vi "PixelLIDAR_Open.vi"() -> (2 "error out":errorcluster, 3 "initialized LIDAR\narray":i32[](array[numeric]), 4 "MDF Image":T1(plugin-control), 5 "MissionMap":path)   [LabVIEW 2012]
doc: "This SubVI sets up the memory space for the Lidars's MDF file and reads the MDF file into it. It is designed to run before Pixel_LIDAR_Run.VI."
panel:
  out "concatenated string":string
  out "Current Path Name":string
  out "Y Resolution":i32
  out "X Resolution":i32
  # "This SubVI is used with PixelLIDAR_Run.VI and reads thw Mission Map file and sets up memory to accomidate it"
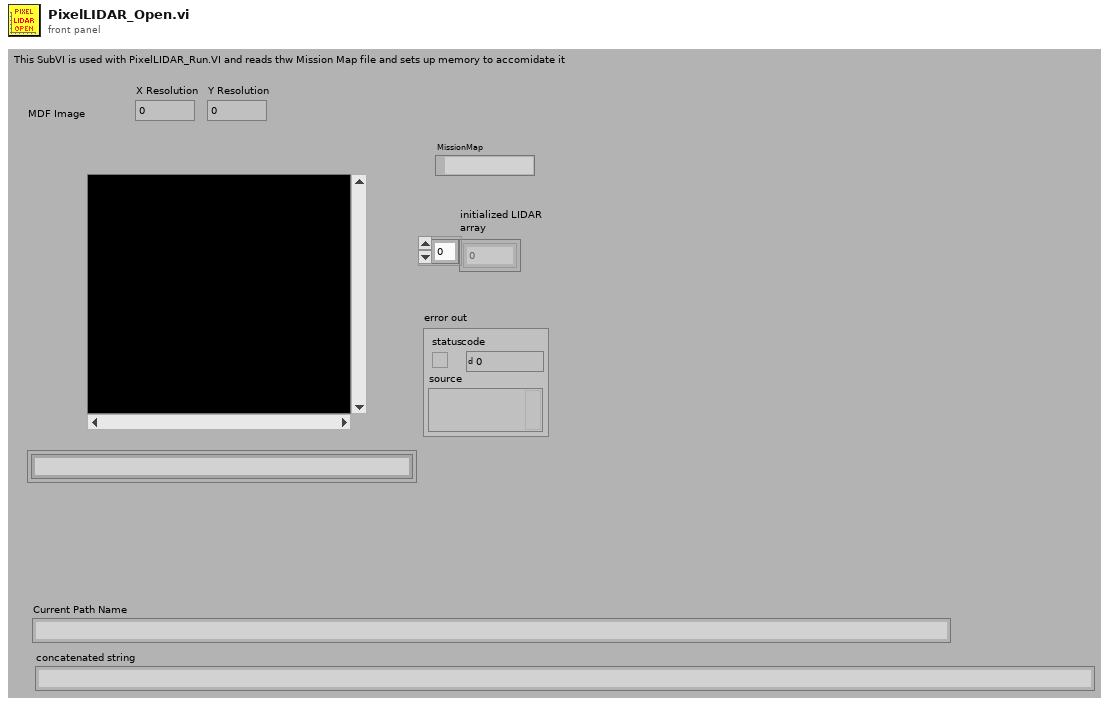
[diagram p1: front panel]
types:
  T1 = typedef "IMAQ Image.ctl" = refnum<image>
  T2 = typedef "Image Type" = u32
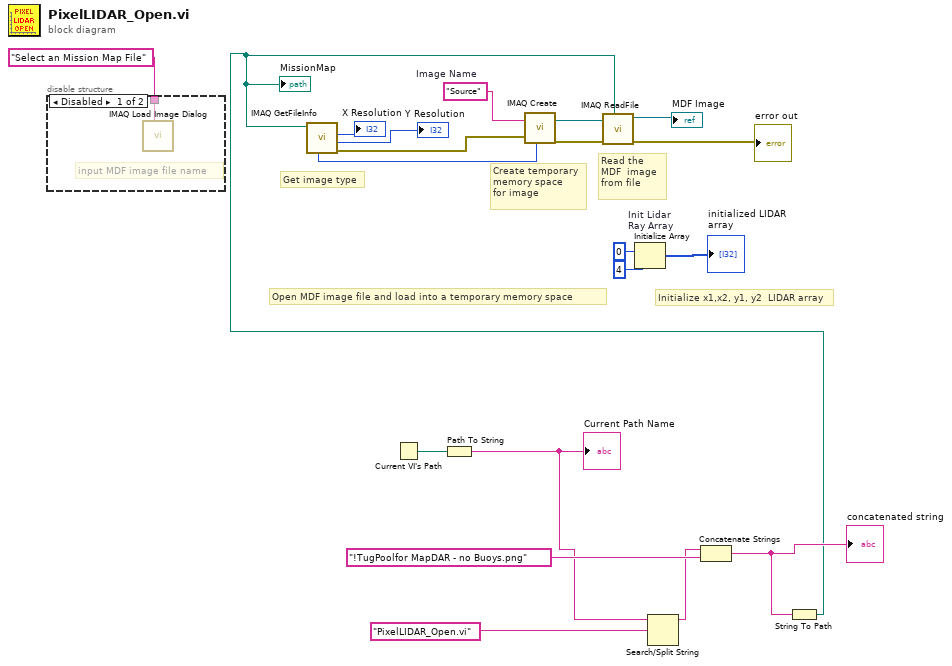
[diagram p0: block diagram]
diagram:
  w17 = "Source"  # Image Name
  # "Initialize x1,x2, y1, y2  LIDAR array"
  # "Get image type"
  # "Read the\nMDF  image\nfrom file"
  # "Create temporary\nmemory space \nfor image"
  # "Open MDF image file and load into a temporary memory space"
  n1 = disable-structure shown="Disabled" {
    disable-tunnel: "Select an Mission Map File" ("prompt") -> [w21 _]
    frame Disabled {
      # "input MDF image file name"
      n2 = call "IMAQ Load Image Dialog"("Prompt"=w21) -> ()  [unwired: 6 in, 5 out]
    }
    frame Enabled {
    }
  }
  n3 = Current VI's Path() -> (path=w7:path)
  n4 = Path To String(path=w7) -> (string=w5:string)
  "Current Path Name" <- w5
  n5 = Initialize Array "Init Lidar\nRay Array"(0 ("element"), 4 ("dimension size")) -> (→"initialized LIDAR\narray":i32[])
  n6 = Search/Split String(string=w5, search string/char (-)="PixelLIDAR_Open.vi" ("Current VI Name")) -> (substring before match=w3:string)  [unwired: 1 in, 2 out]
  n7 = Concatenate Strings(w3, "!TugPoolfor MapDAR - no Buoys.png" ("Image File Name")) -> (w2:string)
  "concatenated string" <- w2
  n8 = String To Path(string=w2) -> (path=w1:path)
  "MissionMap" <- w1
  n9 = call "IMAQ GetFileInfo"("File Path"=w1) -> ("error out"=w18:errorcluster, "Y Resolution"=→"Y Resolution":i32, "X Resolution"=→"X Resolution":i32, "Image Type"=w14:T2)  [unwired: 1 in, 6 out]
  n10 = call "IMAQ Create"("Image Name"=w17, "Image Type"=w14, "error in (no error)"=w18) -> ("New Image"=w19:T1, "error out"=w20:errorcluster)  [unwired: 1 in, 1 out]
  n11 = call "IMAQ ReadFile"("File Path"=w1, "error in (no error)"=w20, "Image"=w19) -> ("error out"=→"error out":errorcluster, "Image Out"=→"MDF Image":T1)  [unwired: 2 in, 5 out]
